vi "Generate New QControl Path.vi"(8 "error in (no error)":errorcluster, 11 "QControl Wizard in":refnum<class "QControl Creation Wizard.lvclass">) -> (0 "error out":errorcluster, 2 "New Class Path":path, 3 "QControl Wizard out":refnum<class "QControl Creation Wizard.lvclass">)   [LabVIEW 2015, in "QControl Creation Wizard.lvclass"]
doc: "<b> </b> <b> </b>\n©2016 Q Software Innovations, LLC (QSI)\nwritten by Quentin Alldredge\nproduced in LabVIEW 2015\n\nsupport@qsoftwareinnovations.com\nwww.qsoftwareinnovations.com\n\nAll rights reserved.\n\nRedistribution and use in source and binary forms, with or without modification, are permitted provided that the following conditions are met:\n\n * Redistributions of source code must retain the above copyright notice, this list of conditions and the following disclaimer.\n * Redistributions in binary form must reproduce the above copyright notice, this list of conditions and the following disclaimer in the documentation and/or other materials provided with the distribution.\n * Neither the name of Q Software Innovations, LLC. nor the names of its contributors may be used to endorse or promote products derived from this software without specific prior written permission.\n\nTHIS SOFTWARE IS PROVIDED BY THE COPYRIGHT HOLDERS AND CONTRIBUTORS \"AS IS\" AND ANY EXPRESS OR IMPLIED WARRANTIES, INCLUDING, BUT NOT LIMITED TO, THE IMPLIED WARRANTIES OF MERCHANTABILITY AND FITNESS FOR A PARTICULAR PURPOSE ARE DISCLAIMED. IN NO EVENT SHALL THE COPYRIGHT OWNER OR CONTRIBUTORS BE LIABLE FOR ANY DIRECT, INDIRECT, INCIDENTAL, SPECIAL, EXEMPLARY, OR CONSEQUENTIAL DAMAGES (INCLUDING, BUT NOT LIMITED TO, PROCUREMENT OF SUBSTITUTE GOODS OR SERVICES; LOSS OF USE, DATA, OR PROFITS; OR BUSINESS INTERRUPTION) HOWEVER CAUSED AND ON ANY THEORY OF LIABILITY, WHETHER IN CONTRACT, STRICT LIABILITY, OR TORT (INCLUDING NEGLIGENCE OR OTHERWISE) ARISING IN ANY WAY OUT OF THE USE OF THIS SOFTWARE, EVEN IF ADVISED OF THE POSSIBILITY OF SUCH DAMAGE."
uses:
  QControl Creation Wizard.lvclass
  QControl Creation Wizard.lvclass/QControl Creation Wizard.ctl
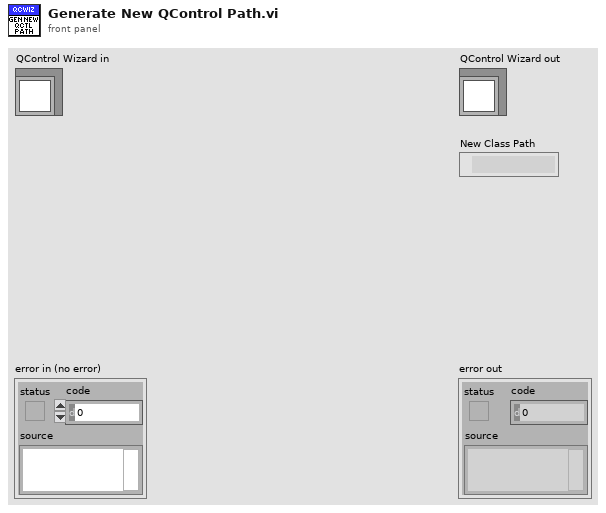
[diagram p1: front panel]
types:
  T1 = enum16{"Don't Add", "To Target", "To Project Item"}
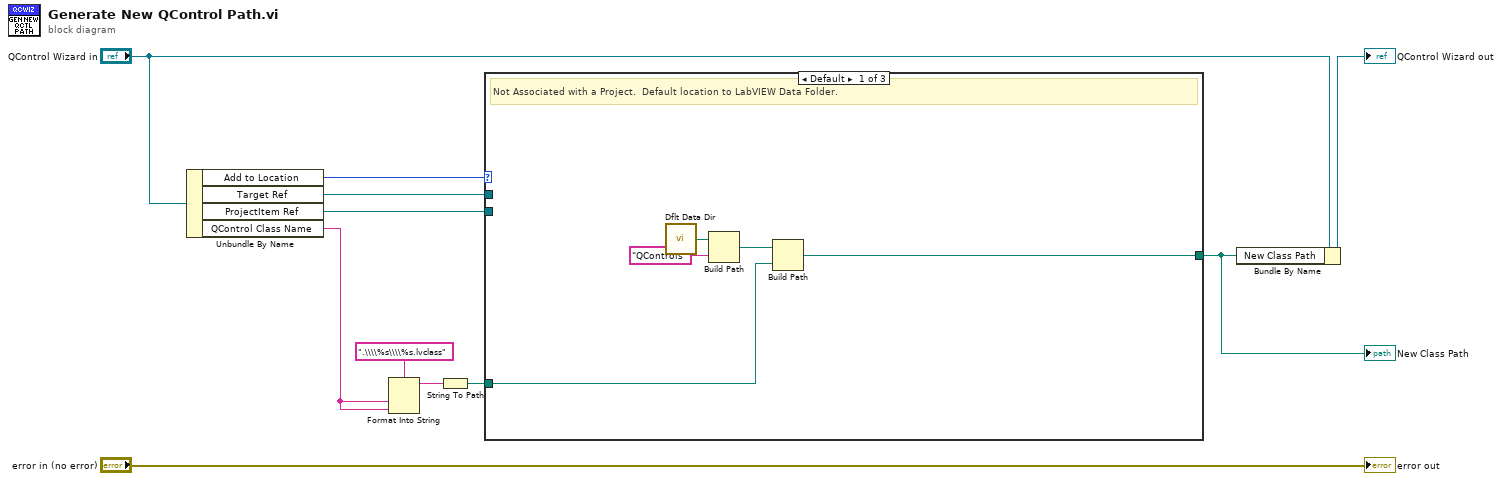
[diagram p0: block diagram]
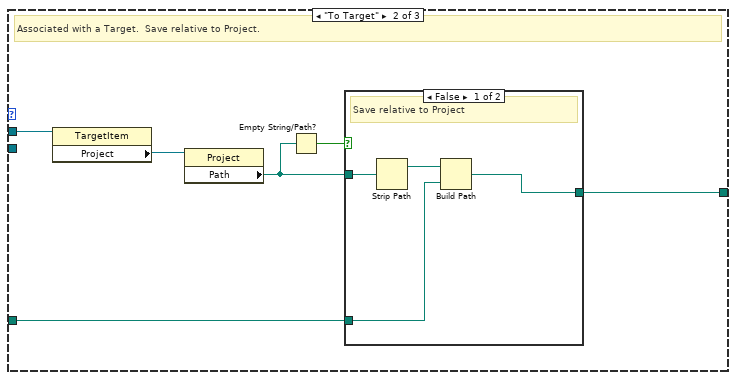
[diagram p2: hidden frame]
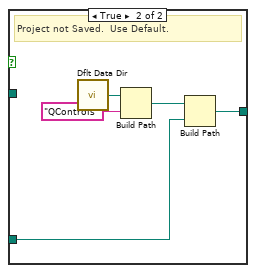
[diagram p3: hidden frame]
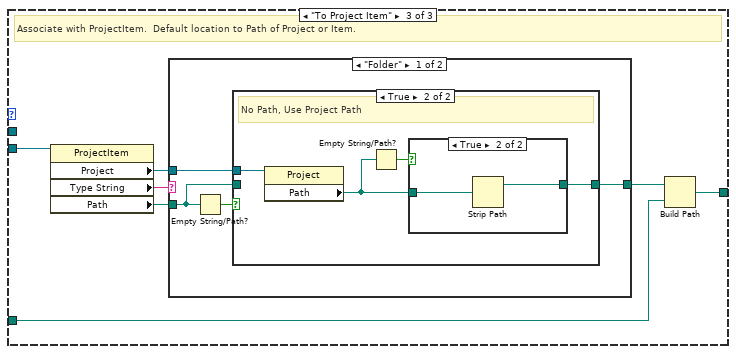
[diagram p4: hidden frame]
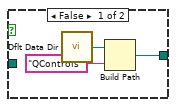
[diagram p6: hidden frame]
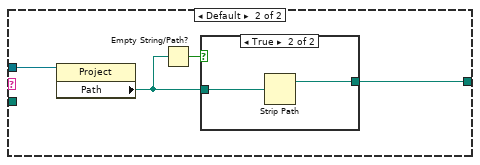
[diagram p7: hidden frame]
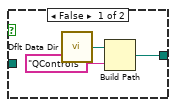
[diagram p8: hidden frame]
diagram:
  n1 = Unbundle By Name("QControl Wizard in") -> ("Add to Location"=w5:T1, "Target Ref"=w3:refnum<vi>, "ProjectItem Ref"=w2:refnum<vi>, "QControl Class Name"=w7:string)
  n2 = Format Into String(format string=".\\\\%s\\\\%s.lvclass", w7, w7) -> (resulting string=w6:string)  [unwired: 2 in, 1 out]
  n3 = String To Path(string=w6) -> (path=w4:path)
  n4 = case shown="Default" w5 {
    tunnel: w4 -> [w12 w20 w37]
    tunnel: w3 -> [_ w22 _]
    tunnel: w2 -> [_ _ w35]
    tunnel: [w13 w19 w36] -> w1
    frame Default {
      # "Not Associated with a Project.  Default location to LabVIEW Data Folder."
      n5 = call <vilib>:"Dflt Data Dir.vi"() -> ("App:Default Data Directory"=w16:path)
      n6 = Build Path(base path=w16, name or relative path="QControls") -> (appended path=w15:path)
      n7 = Build Path(base path=w15, name or relative path=w12) -> (appended path=w13:path)
    }
    frame "To Target" {
      # "Associated with a Target.  Save relative to Project."
      n8 = property class="TargetItem"(reference=w22) -> ("Project"=w21:refnum<vi>)  [unwired: 1 in, 2 out]
      n9 = property class="Project"(reference=w21) -> ("Path"=w18:path)  [unwired: 1 in, 2 out]
      n10 = Empty String/Path?(string/path=w18) -> (empty?=w17:bool)
      n11 = case shown="False" w17 {
        tunnel: w20 -> [w25 w27]
        tunnel: [w24 w28] -> w19
        tunnel: w18 -> [w23 _]
        frame False {
          # "Save relative to Project"
          n12 = Strip Path(path=w23) -> (stripped path=w26:path)  [unwired: 1 out]
          n13 = Build Path(base path=w26, name or relative path=w25) -> (appended path=w24:path)
        }
        frame True {
          # "Project not Saved.  Use Default."
          n14 = call <vilib>:"Dflt Data Dir.vi"() -> ("App:Default Data Directory"=w31:path)
          n15 = Build Path(base path=w31, name or relative path="QControls") -> (appended path=w30:path)
          n16 = Build Path(base path=w30, name or relative path=w27) -> (appended path=w28:path)
        }
      }
    }
    frame "To Project Item" {
      # "Associate with ProjectItem.  Default location to Path of Project or Item."
      n17 = property class="ProjectItem"(reference=w35) -> ("Project"=w33:refnum<vi>, "Type String"=w34:string, "Path"=w32:path)  [unwired: 1 in, 2 out]
      n18 = case shown="\"Folder\"" w34 {
        tunnel: [w40 w53] -> w38
        tunnel: w33 -> [w41 w56]
        tunnel: w32 -> [w39 _]
        frame "Folder" {
          n19 = Empty String/Path?(string/path=w39) -> (empty?=w42:bool)
          n20 = case shown="True" w42 {
            tunnel: w41 -> [_ w47]
            tunnel: [w43 w46] -> w40
            tunnel: w39 -> [w43 _]
            frame False {
              # "Use Folder Path"
            }
            frame True {
              # "No Path, Use Project Path"
              n21 = property class="Project"(reference=w47) -> ("Path"=w45:path)  [unwired: 1 in, 2 out]
              n22 = Empty String/Path?(string/path=w45) -> (empty?=w44:bool)
              n23 = case shown="True" w44 {
                tunnel: w45 -> [_ w52]
                tunnel: [w48 w51] -> w46
                frame False {
                  n24 = call <vilib>:"Dflt Data Dir.vi"() -> ("App:Default Data Directory"=w50:path)
                  n25 = Build Path(base path=w50, name or relative path="QControls") -> (appended path=w48:path)
                }
                frame True {
                  n26 = Strip Path(path=w52) -> (stripped path=w51:path)  [unwired: 1 out]
                }
              }
            }
          }
        }
        frame Default {
          n27 = property class="Project"(reference=w56) -> ("Path"=w54:path)  [unwired: 1 in, 2 out]
          n28 = Empty String/Path?(string/path=w54) -> (empty?=w55:bool)
          n29 = case shown="True" w55 {
            tunnel: w54 -> [_ w61]
            tunnel: [w57 w60] -> w53
            frame False {
              n30 = call <vilib>:"Dflt Data Dir.vi"() -> ("App:Default Data Directory"=w59:path)
              n31 = Build Path(base path=w59, name or relative path="QControls") -> (appended path=w57:path)
            }
            frame True {
              n32 = Strip Path(path=w61) -> (stripped path=w60:path)  [unwired: 1 out]
            }
          }
        }
      }
      n33 = Build Path(base path=w38, name or relative path=w37) -> (appended path=w36:path)
    }
  }
  "New Class Path" <- w1
  n34 = Bundle By Name(cluster="QControl Wizard in", "New Class Path"=w1) -> (→"QControl Wizard out":refnum<class "QControl Creation Wizard.lvclass">)
  "error out" <- "error in (no error)"
